vi "SAW bandwidth.vi"(8 "x array":dbl[](array[numeric]), 9 "best fit y":dbl[](array[numeric]), 11 "best fit parms":dbl[](array[numeric])) -> (0 "Q factor":dbl, 1 "Bandwidth":dbl, 2 "S11 dip":dbl, 3 "fc from fit":dbl)   [LabVIEW 2020]
panel:
  # "Gives best fit parms for S in dB once fitted to lorentzian"
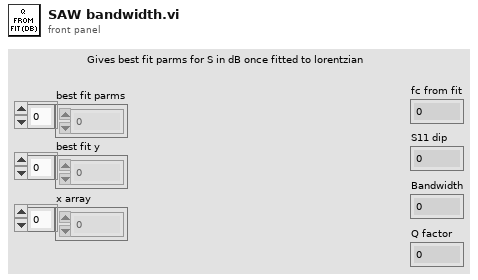
[diagram p1: front panel]
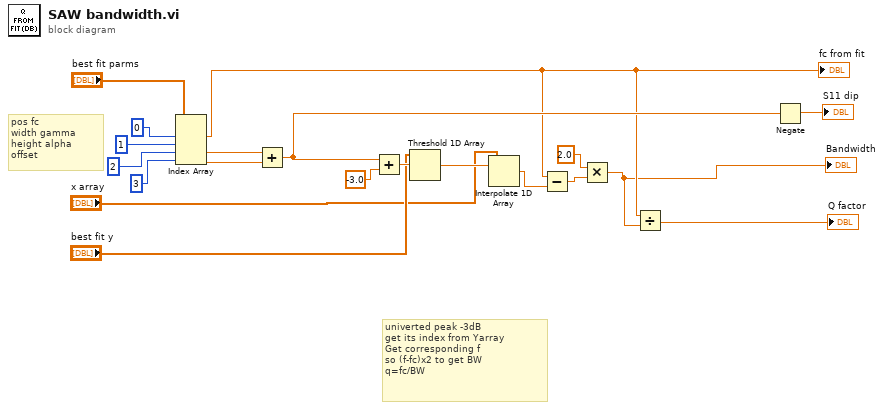
[diagram p0: block diagram]
diagram:
  # "pos fc\nwidth gamma\nheight alpha\noffset"
  # "univerted peak -3dB\nget its index from Yarray\nGet corresponding f\nso (f-fc)x2 to get BW\nq=fc/BW"
  n1 = Index Array(array="best fit parms", index #1=0 ("index"), index #2=1 ("index"), index #3=2 ("index"), index #4=3 ("index")) -> (element #1=w7:dbl, element #3=w16:dbl, element #4=w15:dbl)  [unwired: 1 out]
  "fc from fit" <- w7
  n2 = Add(x=w16, y=w15) -> (x+y=w13:dbl)
  n3 = Add(x=w13, y=-3.0) -> (x+y=w14:dbl)
  n4 = Threshold 1D Array(2:w14, 3:"best fit y") -> (0:w4:dbl)  [unwired: 1 in]
  n5 = Interpolate 1D Array(1:w4, 2:"x array") -> (0:w2:dbl)
  n6 = Subtract(x=w7, y=w2) -> (x-y=w5:dbl)
  n7 = Multiply(x=2.0, y=w5) -> (x*y=w1:dbl)
  "Bandwidth" <- w1
  n8 = Divide(x=w7, y=w1) -> (x/y=→"Q factor":dbl)
  n9 = Negate(x=w13) -> (-x=→"S11 dip":dbl)
